vi "Log Data.vi"(8 "error in (no error)":errorcluster, 10 "Data Queue":refnum<queue>, 11 "Logging Configuration":T1) -> (0 "error out":errorcluster)   [LabVIEW 2014, in "PLS Logging.lvlib"]
doc: "This VI uses the TDMS Write function to write data to a TDMS file."
uses:
  PLS Logging.lvlib
  Logging Configuration.ctl
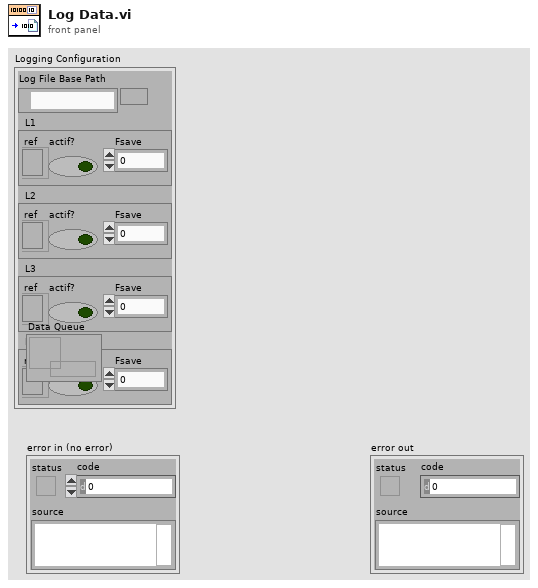
[diagram p1: front panel]
types:
  T1 = typedef "PLS Logging.lvlib/Logging Configuration.ctl" = cluster{"Log File Base Path":path, "L1":cluster{"ref":refnum<file>, "actif?":bool, "Fsave":i32}, "L2":cluster{"ref":refnum<file>, "actif?":bool, "Fsave":i32}, "L3":cluster{"ref":refnum<file>, "actif?":bool, "Fsave":i32}, "L4":cluster{"ref":refnum<file>, "actif?":bool, "Fsave":i32}}
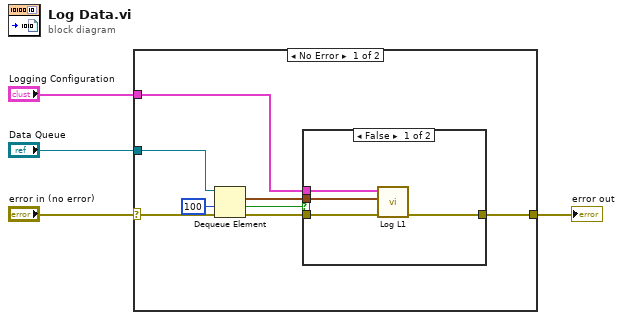
[diagram p0: block diagram]
diagram:
  n1 = case shown="No Error" "error in (no error)" {
    selector: "error in (no error)" -> [w12 w18]
    tunnel: "Logging Configuration" -> [w5 _]
    tunnel: "Data Queue" -> [w11 _]
    tunnel: [w9 w18] -> w2
    frame No Error {
      n2 = Dequeue Element(queue=w11, timeout in ms (-1)=100, error in (no error)=w12) -> (element=w8:waveform(dbl)[], timed out?=w6:bool, error out=w10:errorcluster)  [unwired: 1 out]
      n3 = case shown="False" w6 {
        tunnel: w5 -> [w16 _]
        tunnel: w10 -> [w15 w17]
        tunnel: [w14 w17] -> w9
        tunnel: w8 -> [w13 _]
        frame False {
          n4 = call "Log L1.vi"("error in (no error)"=w15, "Array"=w13, "Logging Configuration"=w16) -> ("error out"=w14:errorcluster)  [unwired: 8 in]
        }
        frame True {
        }
      }
    }
    frame Error {
    }
  }
  "error out" <- w2
